vi "Remove NCoincs present in Coincs.vi"(10 "NCoincs":u64[](array[numeric]), 11 "Coincs":u64[](array[numeric])) -> (3 "NCoincs cleaned":u64[](array[numeric]))   [LabVIEW 2016]
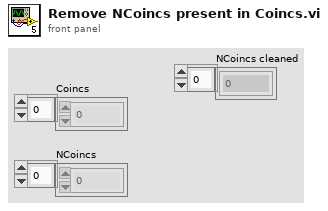
[diagram p1: front panel]
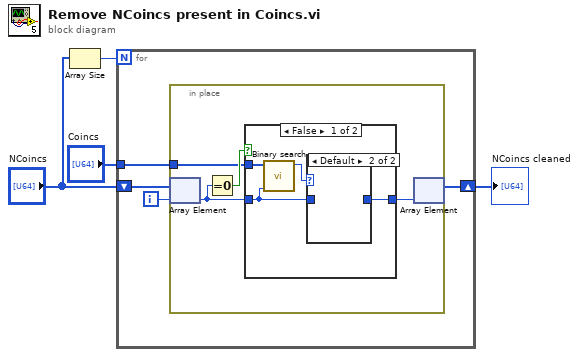
[diagram p0: block diagram]
diagram:
  n1 = Array Size(array="NCoincs") -> (size(s)=w2:i32)
  n2 = for {
    N: w2 -> [_]
    tunnel: "Coincs" -> [w8]
    shift-right: [w5] -> w1
    shift-left: "NCoincs" -> [w7]
    i -> [w6]
    n3 = in-place {
      in-place-border: w8 -> [w9]
      n4 = in-place-array #1(w7, w6) -> (w10:u64)
      n5 = Equal To 0?(x=w10) -> (x = 0?=w12:bool)
      n6 = case shown="False" w12 {
        tunnel: [w16 _] -> w11
        tunnel: w10 -> [w13 _]
        tunnel: w9 -> [w15 _]
        frame False {
          n7 = call "Binary search.vi"("element"=w13, "1D array"=w15) -> ("index"=w14:i32)  [unwired: 9 in]
          n8 = case shown="Default" w14 {
            tunnel: [w17 _] -> w16
            tunnel: w13 -> [w17 _]
            frame -1 {
            }
            frame Default {
            }
          }
        }
        frame True {
        }
      }
      n9 = in-place-array #1(w11) -> (w5:u64[])  [unwired: 1 out]
    }
  }
  "NCoincs cleaned" <- w1
